vi "Py - ZtoName.vi"(7 "python in":refnum<k35>, 8 "error in":errorcluster, 11 "Z":i32) -> (0 "error out":errorcluster, 3 "Element Name":string, 5 "python out":refnum<k35>)   [LabVIEW 2023]
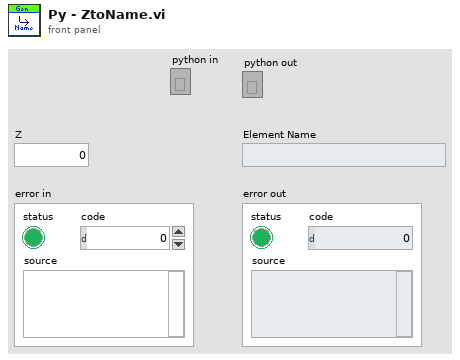
[diagram p1: front panel]
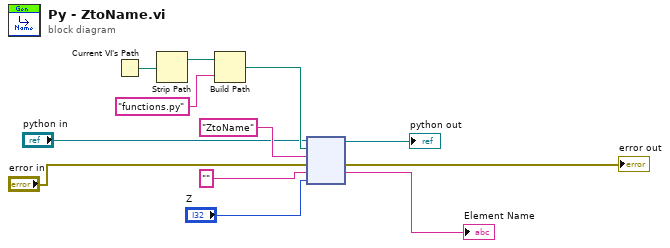
[diagram p0: block diagram]
diagram:
  n1 = Current VI's Path() -> (path=w11:path)
  n2 = Strip Path(path=w11) -> (stripped path=w10:path)  [unwired: 1 out]
  n3 = Build Path(base path=w10, name or relative path="functions.py") -> (appended path=w4:path)
  n4 = node("python in", w4, "ZtoName", "error in", "", "Z") -> (→"python out":refnum<k35>, →"error out":errorcluster, →"Element Name":string)  [unwired: 1 in, 2 out]
